vi "XBee_RX_ADC5.vi"() -> ()   [LabVIEW 2010]
uses:
  <vilib>/Instr/_visa.llb/VISA Configure Serial Port (Instr).vi
panel:
  out "Waveform Chart 4":cluster{dbl}(graph)
  out "ADC 4":dbl=39.0
  out "Waveform Chart 3":cluster{dbl}(graph)
  out "ADC 3":dbl=39.0
  out "Waveform Chart 2":cluster{dbl}(graph)
  out "ADC 2":dbl=39.0
  out "Waveform Chart 1":cluster{dbl}(graph)
  out "ADC 1":dbl=39.0
  out "Waveform Chart":cluster{dbl}(graph)
  out "Sample Quantity":string
  out "Option Byte":string
  out "Start Delimiter":string
  out "CheckSum":dbl=39.0
  out "ADC 0":dbl=39.0
  in  "VISA resource name":refnum<visa-resource-name>="COM4"
  in  "stop":bool
  out "API Packet":string
  out "Channel Indicator":string
  out "Source Address":string="Vx"
  out "Byte Length":dbl=14.0
  out "RSSI":dbl=39.0
  out "API Identifier":dbl=39.0
  in  "byte count":u32=54
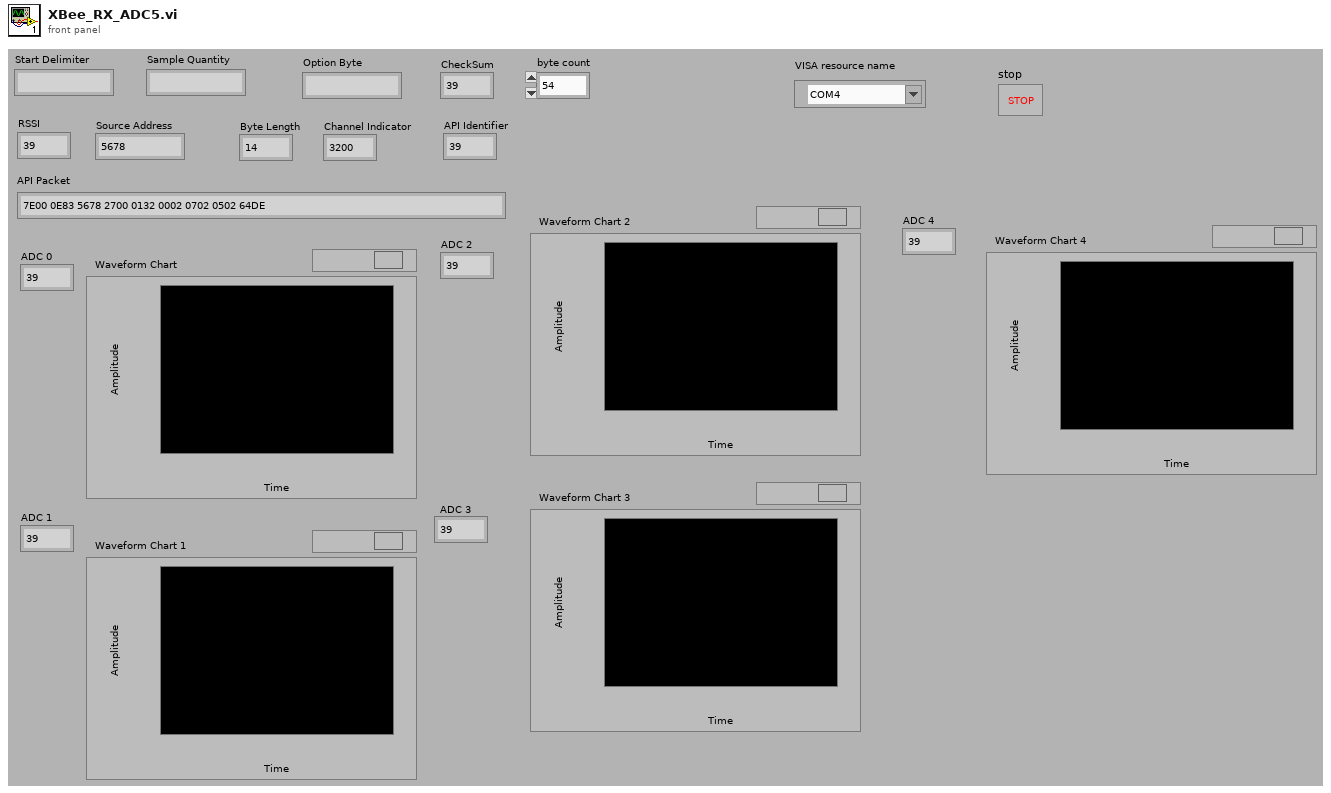
[diagram p1: front panel]
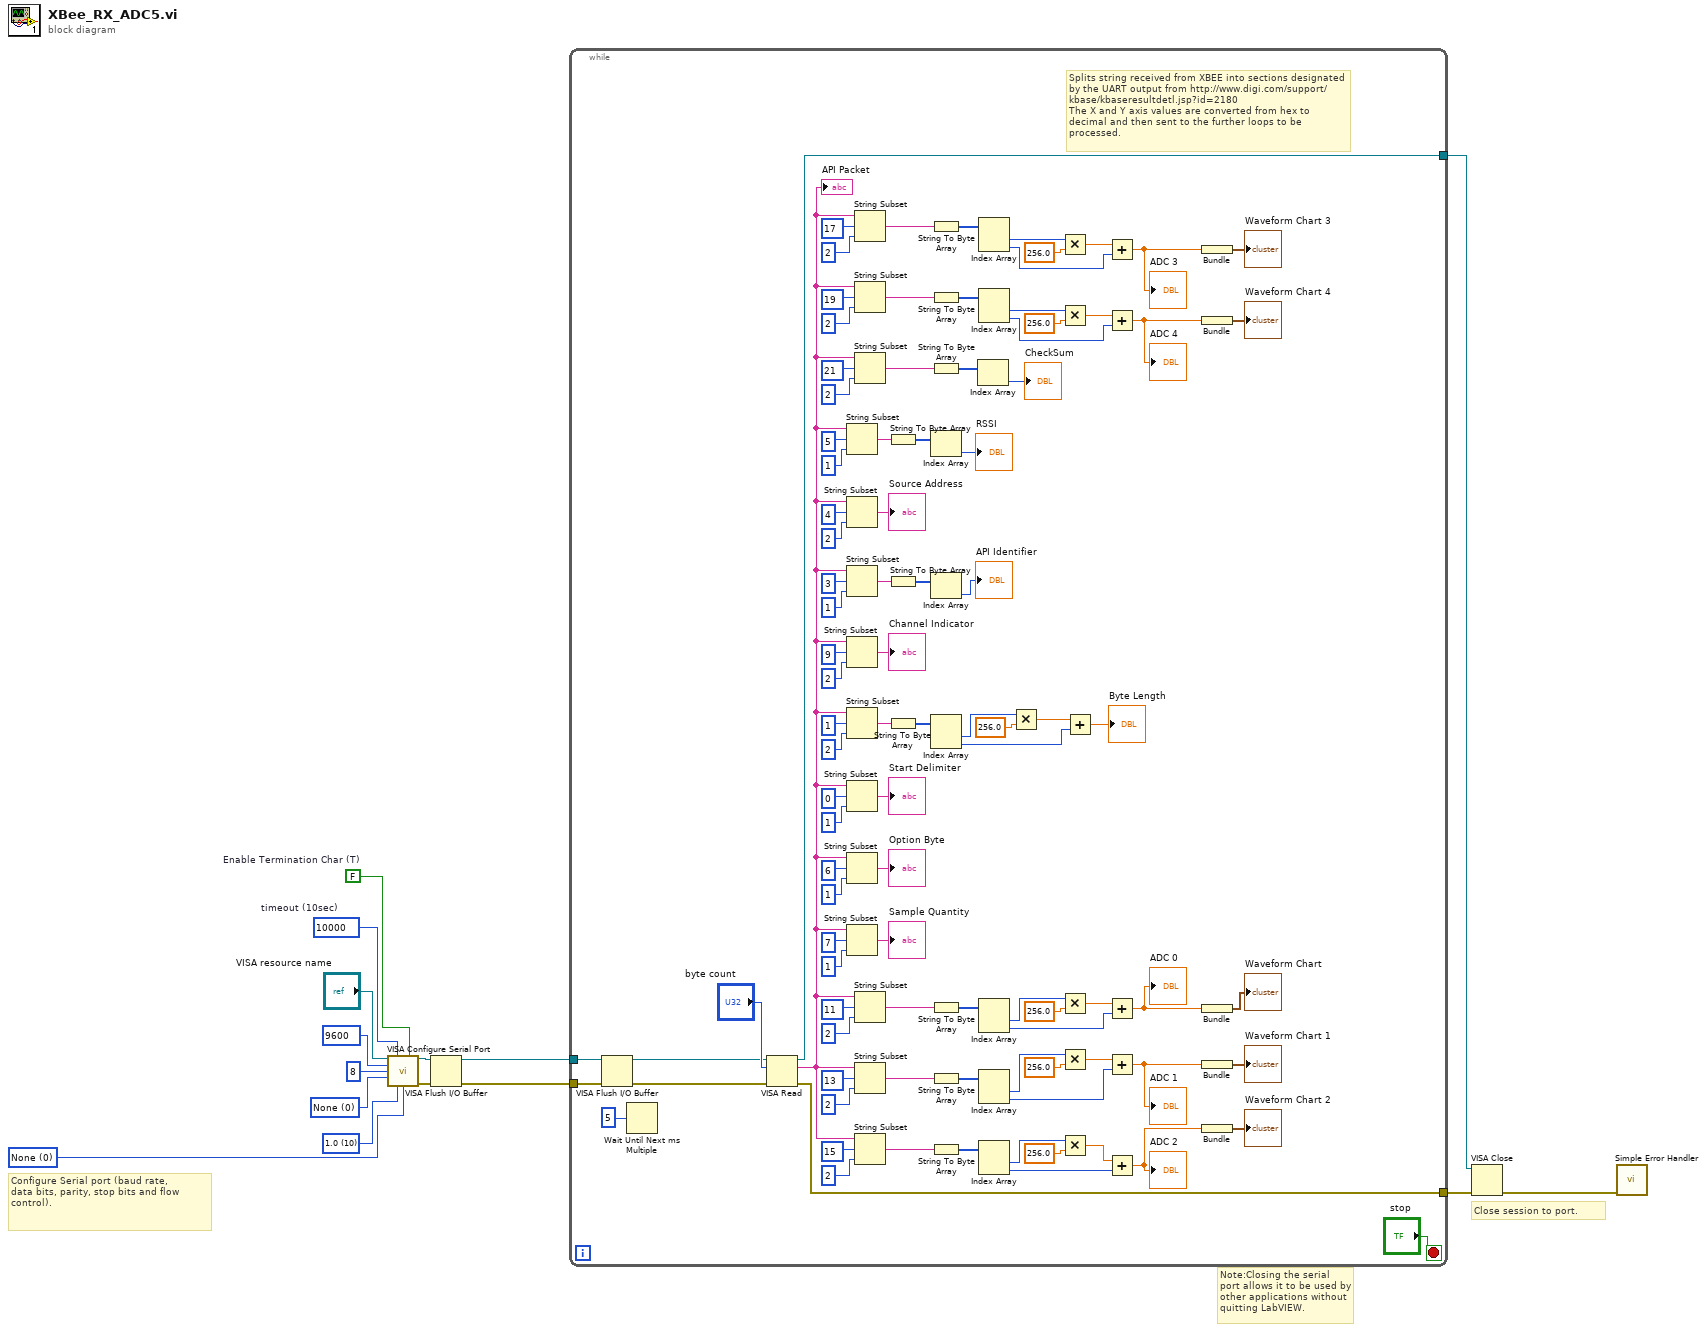
[diagram p0: block diagram]
diagram:
  w4 = u16 0 items=["None"=0, "XON/XOFF"=1, "RTS/CTS"=2, "DTR/DSR"=4] ("flow control")
  w5 = u16 10 items=["1.0"=10, "1.5"=15, "2.0"=20] ("stop bits")
  w8 = u16 0 items=["None", "Odd", "Even", "Mark", "Space"] ("parity")
  w6 = FALSE  # Enable Termination Char (T)
  w7 = u32 10000  # timeout (10sec)
  # "Configure Serial port (baud rate,\ndata bits, parity, stop bits and flow control)."
  # "Note:Closing the serial port allows it to be used by other applications without\nquitting LabVIEW."
  # "Close session to port."
  n1 = call-poly "VISA Configure Serial Port"("VISA resource name"="VISA resource name", "timeout (10sec)"=w7, "Enable Termination\nChar (T)"=w6, "baud rate (9600)"=u32 9600 ("baud rate"), "data bits (8)"=u16 8 ("data bits"), "parity (0:none)"=w8, "stop bits (10: 1 bit)"=w5, "flow control (0:none)"=w4) -> ("VISA resource name out"=w9:refnum<visa-resource-name>, "error out"=w10:errorcluster)  [unwired: 1 in, 5 out]
  n2 = VISA Flush I/O Buffer(VISA resource name=w9, error in (no error)=w10) -> (VISA resource name out=w2:refnum<visa-resource-name>, error out=w1:errorcluster)  [unwired: 1 out]
  n3 = while {
    tunnel: [w114] -> w15
    tunnel: [w113] -> w14
    tunnel: w2 -> [w81]
    tunnel: w1 -> [w82]
    stop <- "stop" stop-if-true
    # "Splits string received from XBEE into sections designated by the UART output from http://www.digi.com/support/kbase/kbaseresultdetl.jsp?id=2180 \nThe X and Y axis values are converted from hex to decimal and then sent to the further loops to be processed."
    n4 = VISA Flush I/O Buffer(VISA resource name=w81, error in (no error)=w82) -> (VISA resource name out=w80:refnum<visa-resource-name>, error out=w79:errorcluster)  [unwired: 1 out]
    n5 = Wait Until Next ms Multiple(millisecond multiple=u32 5 ("milliseconds to wait")) -> ()  [unwired: 1 out]
    n6 = VISA Read(VISA resource name=w80, byte count="byte count", error in (no error)=w79) -> (VISA resource name out=w113:refnum<visa-resource-name>, read buffer=w40:string, error out=w114:errorcluster)  [unwired: 1 out]
    "API Packet" <- w40
    n7 = String Subset(string=w40, offset (0)=5, length (rest)=1 ("length (rest)")) -> (substring=w87:string)
    n8 = String Subset(string=w40, offset (0)=4, length (rest)=2 ("length (rest)")) -> (substring=→"Source Address":string)
    n9 = String Subset(string=w40, offset (0)=3, length (rest)=1 ("length (rest)")) -> (substring=w83:string)
    n10 = String Subset(string=w40, offset (0)=9, length (rest)=2 ("length (rest)")) -> (substring=→"Channel Indicator":string)
    n11 = String Subset(string=w40, offset (0)=1, length (rest)=2 ("length (rest)")) -> (substring=w89:string)
    n12 = String Subset(string=w40, offset (0)=0, length (rest)=1 ("length (rest)")) -> (substring=→"Start Delimiter":string)
    n13 = String Subset(string=w40, offset (0)=6, length (rest)=1 ("length (rest)")) -> (substring=→"Option Byte":string)
    n14 = String Subset(string=w40, offset (0)=7, length (rest)=1 ("length (rest)")) -> (substring=→"Sample Quantity":string)
    n15 = String Subset(string=w40, offset (0)=17, length (rest)=2 ("length (rest)")) -> (substring=w45:string)
    n16 = String Subset(string=w40, offset (0)=19, length (rest)=2 ("length (rest)")) -> (substring=w41:string)
    n17 = String Subset(string=w40, offset (0)=21, length (rest)=2 ("length (rest)")) -> (substring=w63:string)
    n18 = String Subset(string=w40, offset (0)=11, length (rest)=2 ("length (rest)")) -> (substring=w59:string)
    n19 = String Subset(string=w40, offset (0)=13, length (rest)=2 ("length (rest)")) -> (substring=w68:string)
    n20 = String Subset(string=w40, offset (0)=15, length (rest)=2 ("length (rest)")) -> (substring=w49:string)
    n21 = String To Byte Array(string=w87) -> (unsigned byte array=w88:u8[])
    n22 = String To Byte Array(string=w83) -> (unsigned byte array=w84:u8[])
    n23 = String To Byte Array(string=w89) -> (unsigned byte array=w91:u8[])
    n24 = String To Byte Array(string=w45) -> (unsigned byte array=w46:u8[])
    n25 = String To Byte Array(string=w41) -> (unsigned byte array=w42:u8[])
    n26 = String To Byte Array(string=w63) -> (unsigned byte array=w64:u8[])
    n27 = Index Array(array=w88) -> (element=→"RSSI":u8)  [unwired: 1 in]
    n28 = Index Array(array=w84) -> (element=→"API Identifier":u8)  [unwired: 1 in]
    n29 = Index Array(array=w91) -> (element #1=w94:u8, element #2=w92:u8)  [unwired: 2 in]
    n30 = String To Byte Array(string=w59) -> (unsigned byte array=w72:u8[])
    n31 = String To Byte Array(string=w68) -> (unsigned byte array=w69:u8[])
    n32 = String To Byte Array(string=w49) -> (unsigned byte array=w50:u8[])
    n33 = Index Array(array=w64) -> (element=→"CheckSum":u8)  [unwired: 1 in]
    n34 = Index Array(array=w46) -> (element #1=w23:u8, element #2=w22:u8)  [unwired: 2 in]
    n35 = Index Array(array=w42) -> (element #1=w21:u8, element #2=w20:u8)  [unwired: 2 in]
    n36 = Index Array(array=w72) -> (element #1=w56:u8, element #2=w55:u8)  [unwired: 2 in]
    n37 = Index Array(array=w69) -> (element #1=w27:u8, element #2=w26:u8)  [unwired: 2 in]
    n38 = Index Array(array=w50) -> (element #1=w25:u8, element #2=w24:u8)  [unwired: 2 in]
    n39 = Multiply(x=w94, y=256.0) -> (x*y=w93:dbl)
    n40 = Multiply(x=w23, y=256.0) -> (x*y=w32:dbl)
    n41 = Multiply(x=w21, y=256.0) -> (x*y=w29:dbl)
    n42 = Multiply(x=w56, y=256.0) -> (x*y=w57:dbl)
    n43 = Multiply(x=w27, y=256.0) -> (x*y=w38:dbl)
    n44 = Multiply(x=w25, y=256.0) -> (x*y=w35:dbl)
    n45 = Add(x=w93, y=w92) -> (x+y=→"Byte Length":dbl)
    n46 = Add(x=w32, y=w22) -> (x+y=w31:dbl)
    "ADC 3" <- w31
    n47 = Add(x=w29, y=w20) -> (x+y=w28:dbl)
    "ADC 4" <- w28
    n48 = Add(x=w57, y=w55) -> (x+y=w53:dbl)
    "ADC 0" <- w53
    n49 = Add(x=w38, y=w26) -> (x+y=w37:dbl)
    "ADC 1" <- w37
    n50 = Add(x=w35, y=w24) -> (x+y=w34:dbl)
    "ADC 2" <- w34
    n51 = Bundle(w31) -> (→"Waveform Chart 3":cluster{dbl})  [unwired: 1 out]
    n52 = Bundle(w28) -> (→"Waveform Chart 4":cluster{dbl})  [unwired: 1 out]
    n53 = Bundle(w53) -> (→"Waveform Chart":cluster{dbl})  [unwired: 1 out]
    n54 = Bundle(w37) -> (→"Waveform Chart 1":cluster{dbl})  [unwired: 1 out]
    n55 = Bundle(w34) -> (→"Waveform Chart 2":cluster{dbl})  [unwired: 1 out]
  }
  n56 = VISA Close(VISA resource name=w14, error in (no error)=w15) -> (error out=w13:errorcluster)
  n57 = call <vilib>:"Simple Error Handler.vi"("error in (no error)"=w13) -> ()  [unwired: 1 in, 8 out]
